vi "ApplyLayoutToObject.vi"(5 "scaling settings":T1={"scaling factor"={"horizontal"=1.0, "vertical"=1.0}, "scaling to ignore"=variant} {"scaling factor"."vertical" min=0.0; "scaling factor"."horizontal" min=0.0}, 7 "properties to ignore":variant, 8 "error in (no error)":errorcluster, 10 "GObj Refnum":refnum<vi>, 11 "Control Layout in":refnum<class "GraphChart Control Layout.lvclass">) -> (0 "error out":errorcluster, 3 "Control Layout out":refnum<class "GraphChart Control Layout.lvclass">)   [LabVIEW 2010, in "NI_SE_Front Panel Layout.lvlib" / "GraphChart Control Layout.lvclass"]
doc: "Apply layout information to the GObj Refnum."
uses:
  GraphChart Control Layout.lvclass
  Scaling Factor_Options.ctl
  XY Scaling Factor.ctl
  Control Layout/Control Layout.lvclass
  GraphChart Control Layout.lvclass/GraphChart Control Layout.ctl
  NI_SE_Front Panel Layout.lvlib
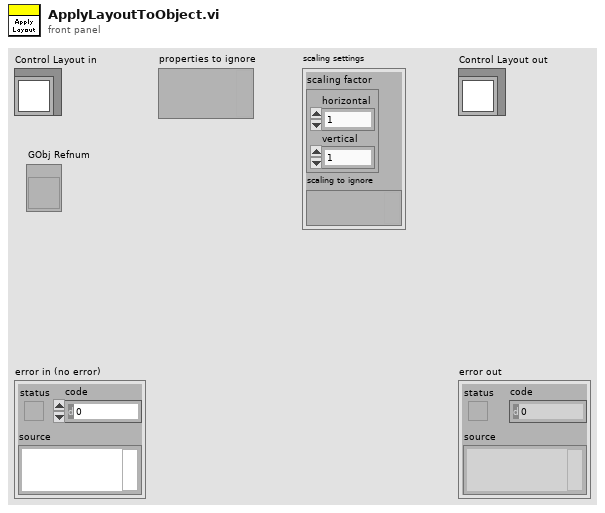
[diagram p1: front panel]
types:
  T1 = typedef "NI_SE_Front Panel Layout.lvlib/Scaling Factor_Options.ctl" = cluster{"scaling factor":T2, "scaling to ignore":variant}
  T2 = typedef "NI_SE_Front Panel Layout.lvlib/XY Scaling Factor.ctl" = cluster{"horizontal":dbl, "vertical":dbl}
  T3 = typedef "LVRectTypeDef.ctl" = cluster{"Left":i16, "Top":i16, "Right":i16, "Bottom":i16}
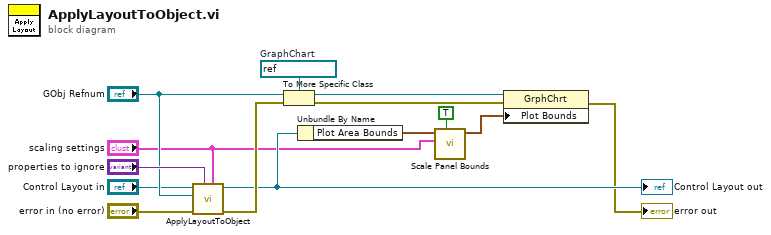
[diagram p0: block diagram]
diagram:
  w6 = refnum<vi> refnum  # GraphChart
  n1 = call-parent "ApplyLayoutToObject.vi"("scaling settings"="scaling settings", "properties to ignore"="properties to ignore", "error in (no error)"="error in (no error)", "GObj Refnum"="GObj Refnum", "Control Layout in"="Control Layout in") -> ("error out"=w11:errorcluster, "Control Layout out"=w9:refnum<class "GraphChart Control Layout.lvclass">)  [unwired: 5 in]
  "Control Layout out" <- w9
  n2 = To More Specific Class(target class=w6, reference="GObj Refnum", error in=w11) -> (specific class reference=w4:refnum<vi>, error out=w5:errorcluster)
  n3 = Unbundle By Name(w9) -> ("Plot Area Bounds"=w3:T3)
  n4 = call "Scale Panel Bounds.vi"("scale position? (F)"=TRUE, "scaling settings"="scaling settings", "bounds in"=w3) -> ("bounds out"=w2:T3)  [unwired: 8 in]
  n5 = property class="GrphChrt"(reference=w4, error in=w5, "Plot Bounds"=w2) -> (error out=→"error out":errorcluster)  [unwired: 1 out]
